vi "SerialNo2.vi"() -> (2 "Continue?":bool)   [LabVIEW 2018]
uses:
  globals/QC_RunInformation.vi
panel:
  in  "Comments:":string
  in  "DB Serial No.:":string
  in  "Batch :":string
  in  "Device Category:":string(combo)="ATLAS18SS"
  in  "Manufacturer:":string(combo)="Hamamatsu"
  in  "Wafer No.:":string
  in  "Cancel":bool
  in  "OK":bool
  in  "Barcode reader":bool
  # "ATLAS Serial No."
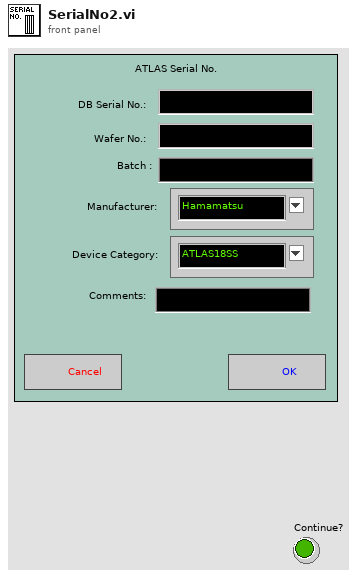
[diagram p1: front panel]
types:
  T1 = cluster{"Institute":string, "Manufacturers":string[], "Devices":string[], "Serialnumbers Lookup DB":string, "Data directory":string, "Backup & screenshot directory":string, "List of known users":string[], "Measurement switch not used":bool, "Measurement Switch":string, "DUT Switch":string, "Rseries IV [MOhm]":string, "Rshunt IV [MOhm]":string, "Rseries CV [MOhm]":string, "DC blocking Cap [µF]":string, "Rseries LCR [MOhm]":string, "Rseries stability [MOhm]":string, "Rshunt stability [MOhm]":string, "Rseries striptest bias [MOhm]":string, "Rseries strip pinhole [MOhm]":string}
  T2 = cluster{"Sensor Serial No.:":string, "Wafer:":string, "Batch:":string, "Manufacturer:":string, "Device Category:":string, "Database Serial No.:":string, "Date Initiated:":string, "Time Initiated:":string, "Test":string, "Probeplan used:":string, "End of Run comment:":string, "User:":string, "Vbias SMU":string, "LCR":string, "Test SMU":string, "Test DMM":string, "Comments":string}
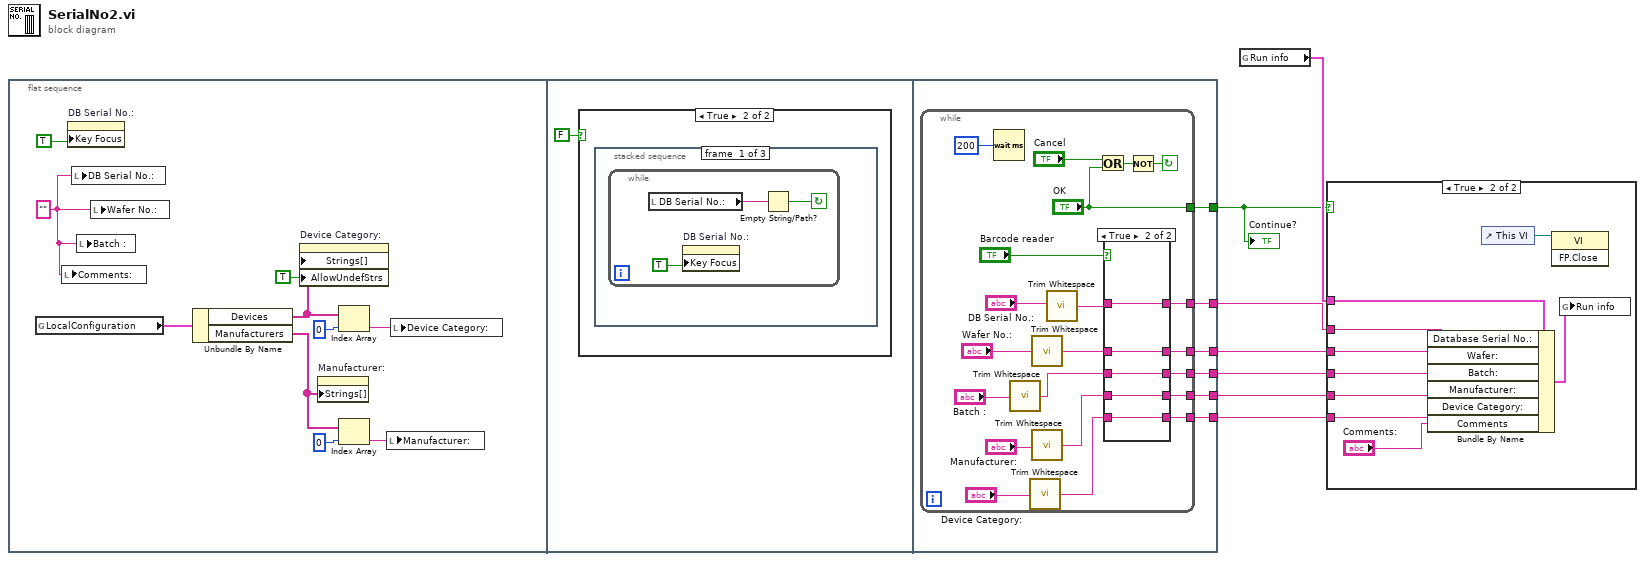
[diagram p0: block diagram]
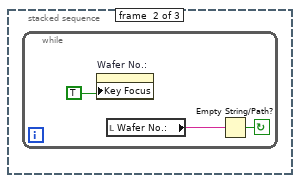
[diagram p4: hidden frame]
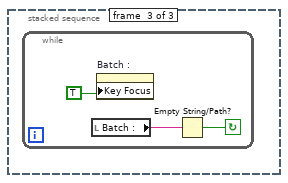
[diagram p5: hidden frame]
diagram:
  n1 = flat-sequence {
    tunnel: [w33] -> w7
    tunnel: [w32] -> w2
    tunnel: [w31] -> w5
    tunnel: [w30] -> w6
    tunnel: [w29] -> w1
    tunnel: [w28] -> w3
    frame #0 {
      w8 = ""
      n2 = global read "QC_RunInformation.vi" "LocalConfiguration"() -> (w16:T1)
      n3 = local write "Comments:"(w8) -> ()
      n4 = property on="DB Serial No.:" class="Str"("Key Focus"=TRUE) -> ()  [unwired: 2 in, 2 out]
      n5 = local write "DB Serial No.:"(w8) -> ()
      n6 = local write "Batch :"(w8) -> ()
      n7 = local write "Wafer No.:"(w8) -> ()
      n8 = Unbundle By Name(w16) -> ("Devices"=w11:string[], "Manufacturers"=w10:string[])
      n9 = property on="Device Category:" class="CmbBox"("Strings[]"=w11, "AllowUndefStrs"=TRUE ("Allow Undefined Strings")) -> ()  [unwired: 2 in, 2 out]
      n10 = property on="Manufacturer:" class="CmbBox"("Strings[]"=w10) -> ()  [unwired: 2 in, 2 out]
      n11 = Index Array(array=w11, index=0) -> (element=w12:string)
      n12 = Index Array(array=w10, index=0) -> (element=w13:string)
      n13 = local write "Manufacturer:"(w13) -> ()
      n14 = local write "Device Category:"(w12) -> ()
    }
    frame #1 {
      n15 = case shown="True" FALSE {
        frame False {
        }
        frame True {
          n16 = stacked-sequence {
            frame #0 {
              n17 = while {
                stop <- w19 continue-if-true
                n18 = local read "DB Serial No.:"() -> (w20:string)
                n19 = property on="DB Serial No.:" class="Str"("Key Focus"=TRUE) -> ()  [unwired: 2 in, 2 out]
                n20 = Empty String/Path?(string/path=w20) -> (empty?=w19:bool)
              }
            }
            frame #1 {
              n21 = while {
                stop <- w23 continue-if-true
                n22 = property on="Wafer No.:" class="Str"("Key Focus"=TRUE) -> ()  [unwired: 2 in, 2 out]
                n23 = local read "Wafer No.:"() -> (w22:string)
                n24 = Empty String/Path?(string/path=w22) -> (empty?=w23:bool)
              }
            }
            frame #2 {
              n25 = while {
                stop <- w26 continue-if-true
                n26 = local read "Batch :"() -> (w25:string)
                n27 = property on="Batch :" class="Str"("Key Focus"=TRUE) -> ()  [unwired: 2 in, 2 out]
                n28 = Empty String/Path?(string/path=w25) -> (empty?=w26:bool)
              }
            }
          }
        }
      }
    }
    frame #2 {
      n29 = while {
        tunnel: ["OK"] -> w32
        tunnel: [w47] -> w29
        tunnel: [w48] -> w33
        tunnel: [w46] -> w28
        tunnel: [w45] -> w31
        tunnel: [w44] -> w30
        stop <- w52 continue-if-true
        n30 = Wait (ms)(milliseconds to wait=200) -> ()  [unwired: 1 out]
        n31 = call <vilib>:"Trim Whitespace.vi"("string"="Batch :") -> ("trimmed string"=w38:string)  [unwired: 1 in]
        n32 = call <vilib>:"Trim Whitespace.vi"("string"="Device Category:") -> ("trimmed string"=w34:string)  [unwired: 1 in]
        n33 = call <vilib>:"Trim Whitespace.vi"("string"="Wafer No.:") -> ("trimmed string"=w40:string)  [unwired: 1 in]
        n34 = call <vilib>:"Trim Whitespace.vi"("string"="Manufacturer:") -> ("trimmed string"=w36:string)  [unwired: 1 in]
        n35 = call <vilib>:"Trim Whitespace.vi"("string"="DB Serial No.:") -> ("trimmed string"=w42:string)  [unwired: 1 in]
        n36 = Or(x="Cancel", y="OK") -> (x .or. y?=w53:bool)
        n37 = case shown="True" "Barcode reader" {
          tunnel: w42 -> [w59 w64]
          tunnel: w40 -> [w58 w63]
          tunnel: [w59 w64] -> w48
          tunnel: [w58 w63] -> w47
          tunnel: w38 -> [w57 w62]
          tunnel: [w57 w62] -> w46
          tunnel: w36 -> [w56 w61]
          tunnel: [w56 w61] -> w45
          tunnel: w34 -> [w55 w60]
          tunnel: [w55 w60] -> w44
          frame False {
          }
          frame True {
          }
        }
        n38 = Not(x=w53) -> (.not. x?=w52:bool)
      }
    }
  }
  n39 = global read "QC_RunInformation.vi" "Run info"() -> (w4:T2)
  n40 = case shown="True" w2 {
    tunnel: w7 -> [_ w73]
    tunnel: w6 -> [_ w72]
    tunnel: w5 -> [_ w71]
    tunnel: w4 -> [_ w70]
    tunnel: w3 -> [_ w69]
    tunnel: w1 -> [_ w67]
    frame False {
    }
    frame True {
      n41 = Bundle By Name(cluster=w70, "Database Serial No.:"=w73, "Wafer:"=w67, "Batch:"=w69, "Manufacturer:"=w71, "Device Category:"=w72, "Comments"="Comments:") -> (w68:T2)
      n42 = control-ref of="This VI"() -> (w66:refnum<vi>)
      n43 = invoke class="VI" method="FP.Close"(reference=w66) -> ()  [unwired: 2 in, 3 out]
      n44 = global write "QC_RunInformation.vi" "Run info"(w68) -> ()
    }
  }
  "Continue?" <- w2
